vi "ASI_Ctrl_Index.vi"(8 "NewVal":variant, 9 "OldVal":variant) -> (2 "ASI out":T1 {"Velocity" min=0.001; "F (um)" min=0.001; "Z (um)" min=0.001; "Step Size (um)" min=0.001}, 3 "Control Ref OUT":refnum<vi>)   [LabVIEW 2014]
uses:
  Type Defs/ASI.ctl
panel:
  in  "ASI in":T1 {"Velocity" min=0.001; "F (um)" min=0.001; "Z (um)" min=0.001; "Step Size (um)" min=0.001}
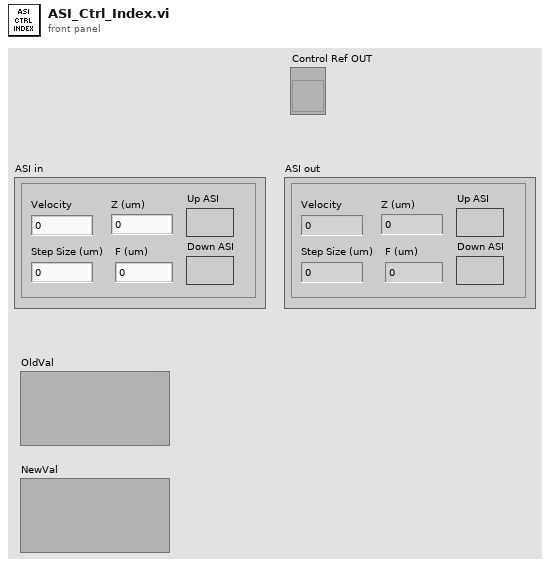
[diagram p1: front panel]
types:
  T1 = typedef "ASI.ctl" = cluster{"Up ASI":bool, "Down ASI":bool, "Step Size (um)":dbl, "Z (um)":dbl, "F (um)":dbl, "Velocity":dbl}
  T2 = cluster{"Up ASI":bool, "Down ASI":bool, "Step Size (um)":bool, "Z (um)":bool, "F (um)":bool, "Velocity":bool}
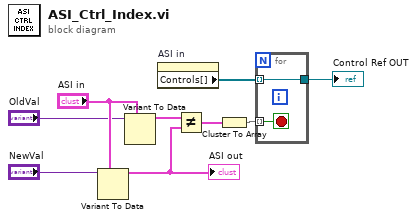
[diagram p0: block diagram]
diagram:
  n1 = Variant To Data(type="ASI in", Variant="NewVal") -> (data=w8:T1)  [unwired: 1 in, 1 out]
  "ASI out" <- w8
  n2 = Variant To Data(type="ASI in", Variant="OldVal") -> (data=w3:T1)  [unwired: 1 in, 1 out]
  n3 = property on="ASI in" class="Clust"() -> ("Controls[]"=w1:refnum<vi>[])  [unwired: 2 in, 2 out]
  n4 = Not Equal?(x=w3, y=w8) -> (x != y?=w7:T2)
  n5 = Cluster To Array(cluster=w7) -> (array=w4:bool[])
  n6 = for {
    tunnel: w4 -> [w10] mode=indexing
    tunnel: w1 -> [w11] mode=indexing
    tunnel: [w11] -> w2
    stop <- w10 stop-if-true
  }
  "Control Ref OUT" <- w2
